vi "DAQ Test Program.vi"(8 "error in (no error)":errorcluster) -> (0 "error out":errorcluster)   [LabVIEW 2018, in "DAQ.lvlib"]
uses:
  DAQ.lvlib
  Acquisition/Acquisition State.ctl
  <vilib>/Platform/TimedLoop/XDataNode/timing_clust.ctl
  <vilib>/Platform/TimedLoop/XDataNode/nitl_modes.ctl
  <vilib>/Platform/TimedLoop/XDataNode/wakeup.ctl
  Acquisition/Task Cluster.ctl
  Acquisition/Hardware Configuration.ctl
  controls/Queue and Message Cluster.ctl
  support/Message Queue/Message Cluster.ctl
  support/Message Queue/Enqueue Message (Single).vi
  <vilib>/Platform/TimedLoop/XDataNode/XDataNode.xnode
  DAQ Write Folder/DAQ/DAQ Write.lvlib
  support/Message Queue/Message Queue.lvlib
  Report Generation/Report Generation.lvlib
  Acquisition/Acquisition Settings Dialog.vi
  support/Support Library.lvlib
  <vilib>/Platform/TimedLoop/XDataNode/XDNodeRunTimeDep.lvlib
panel:
  out "error IO":errorcluster
  out "Data Cluster 2":T1
  out "Task D-O Channels":string[][](array[string])
  in  "Stop Button":bool
  in  "Start Button":bool
  in  "Data Cluster":T1
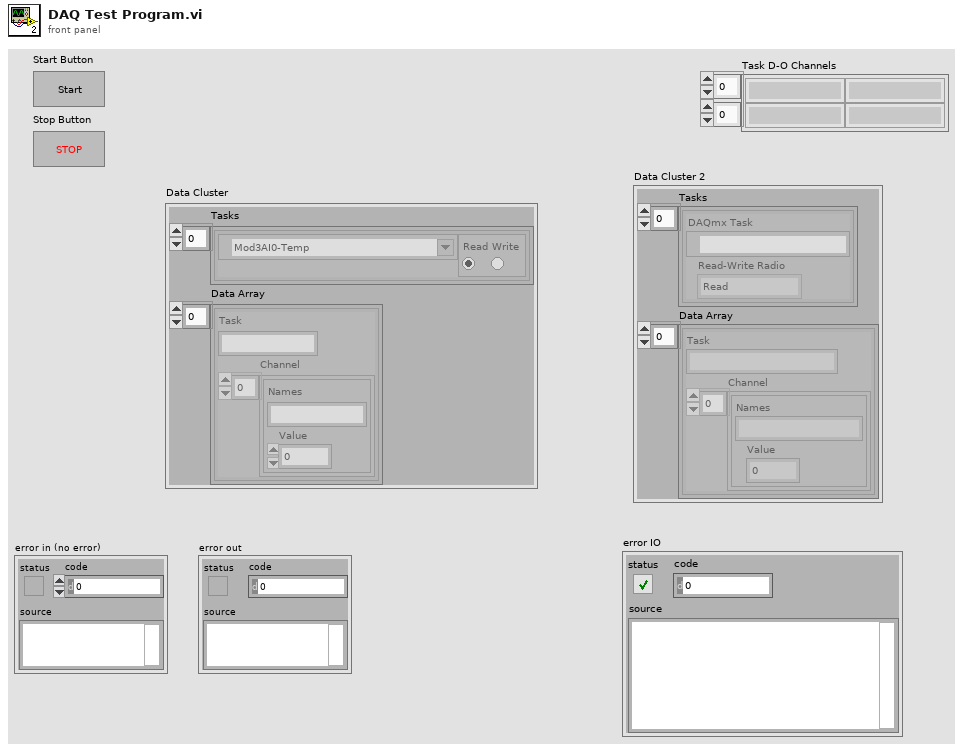
[diagram p1: front panel]
types:
  T1 = cluster{"Tasks":cluster{"DAQmx Task":refnum<k21>, "Read-Write Radio":enum32{"Read", "Write"}}[], "Data Array":cluster{"Task":string, "Channel":cluster{"Names":string, "Value":dbl}[]}[]}
  T2 = typedef "XDNodeRunTimeDep.lvlib/timing_clust.ctl" = cluster{"Expected End [f-1]":u64, "Actual End [f-1]":u64, "Finished Late? [f-1]":bool, "Expected End [i-1]":u64, "Actual End [i-1]":u64, "Finished Late? [i-1]":bool, "Expected Start [i]":u64, "Actual Start [i]":u64, "Expected Start [f]":u64, "Actual Start [f]":u64, "Source Name":string, "Structure Name":string, "Period":i64, "Deadline":i64, "Offset":i64, "Start":i64, "Priority":i32, "Timeout":i32, "Mode":T3, "Wakeup Reason":T4, "Error":errorcluster, "Source Type":string, "Secondary Source Type":string, "Global End Time":u64, "Global Start Time":u64, "Frame Duration":u64, "Iteration Duration":u64, "Assigned CPU":i32, "I/O Scan Engine Mode":u32}
  T3 = typedef "XDNodeRunTimeDep.lvlib/nitl_modes.ctl" = enum32{"No Change", "Process missed periods, maintain original phase", "Discard missed periods, maintain original phase", "Process missed periods, ignore original phase", "Discard missed periods, ignore original phase"}
  T4 = typedef "XDNodeRunTimeDep.lvlib/wakeup.ctl" = enum32{"Normal", "Aborted", "Asynchronous wakeup", "Timing source error", "Timed loop error", "Timeout"}
  T5 = typedef "Task Cluster.ctl" = cluster{"DAQmx Task":refnum<k21>, "Read-Write Radio":enum32{"Read", "Write"}}
  T6 = typedef "DAQ.lvlib/Hardware Configuration.ctl" = cluster{"Tasks Array":T5[]}
  T7 = typedef "DAQ.lvlib/DAQ Write.lvlib/Acquisition State.ctl" = enum16{"Idle", "Acquiring"}
  T8 = typedef "Queue and Message Cluster.ctl" = cluster{"return Message Queue":refnum<queue>, "Message":string, "Variant":variant}
  T9 = cluster{"DAQmx Task":refnum<k21>, "Read-Write Radio":enum32{"Read", "Write"}}[]
  T10 = cluster{"Task":string, "Channel":cluster{"Names":string, "Value":dbl}[]}[]
  T11 = typedef "Message Queue.lvlib/Message Cluster.ctl" = cluster{"Message":string, "Message Data":variant}
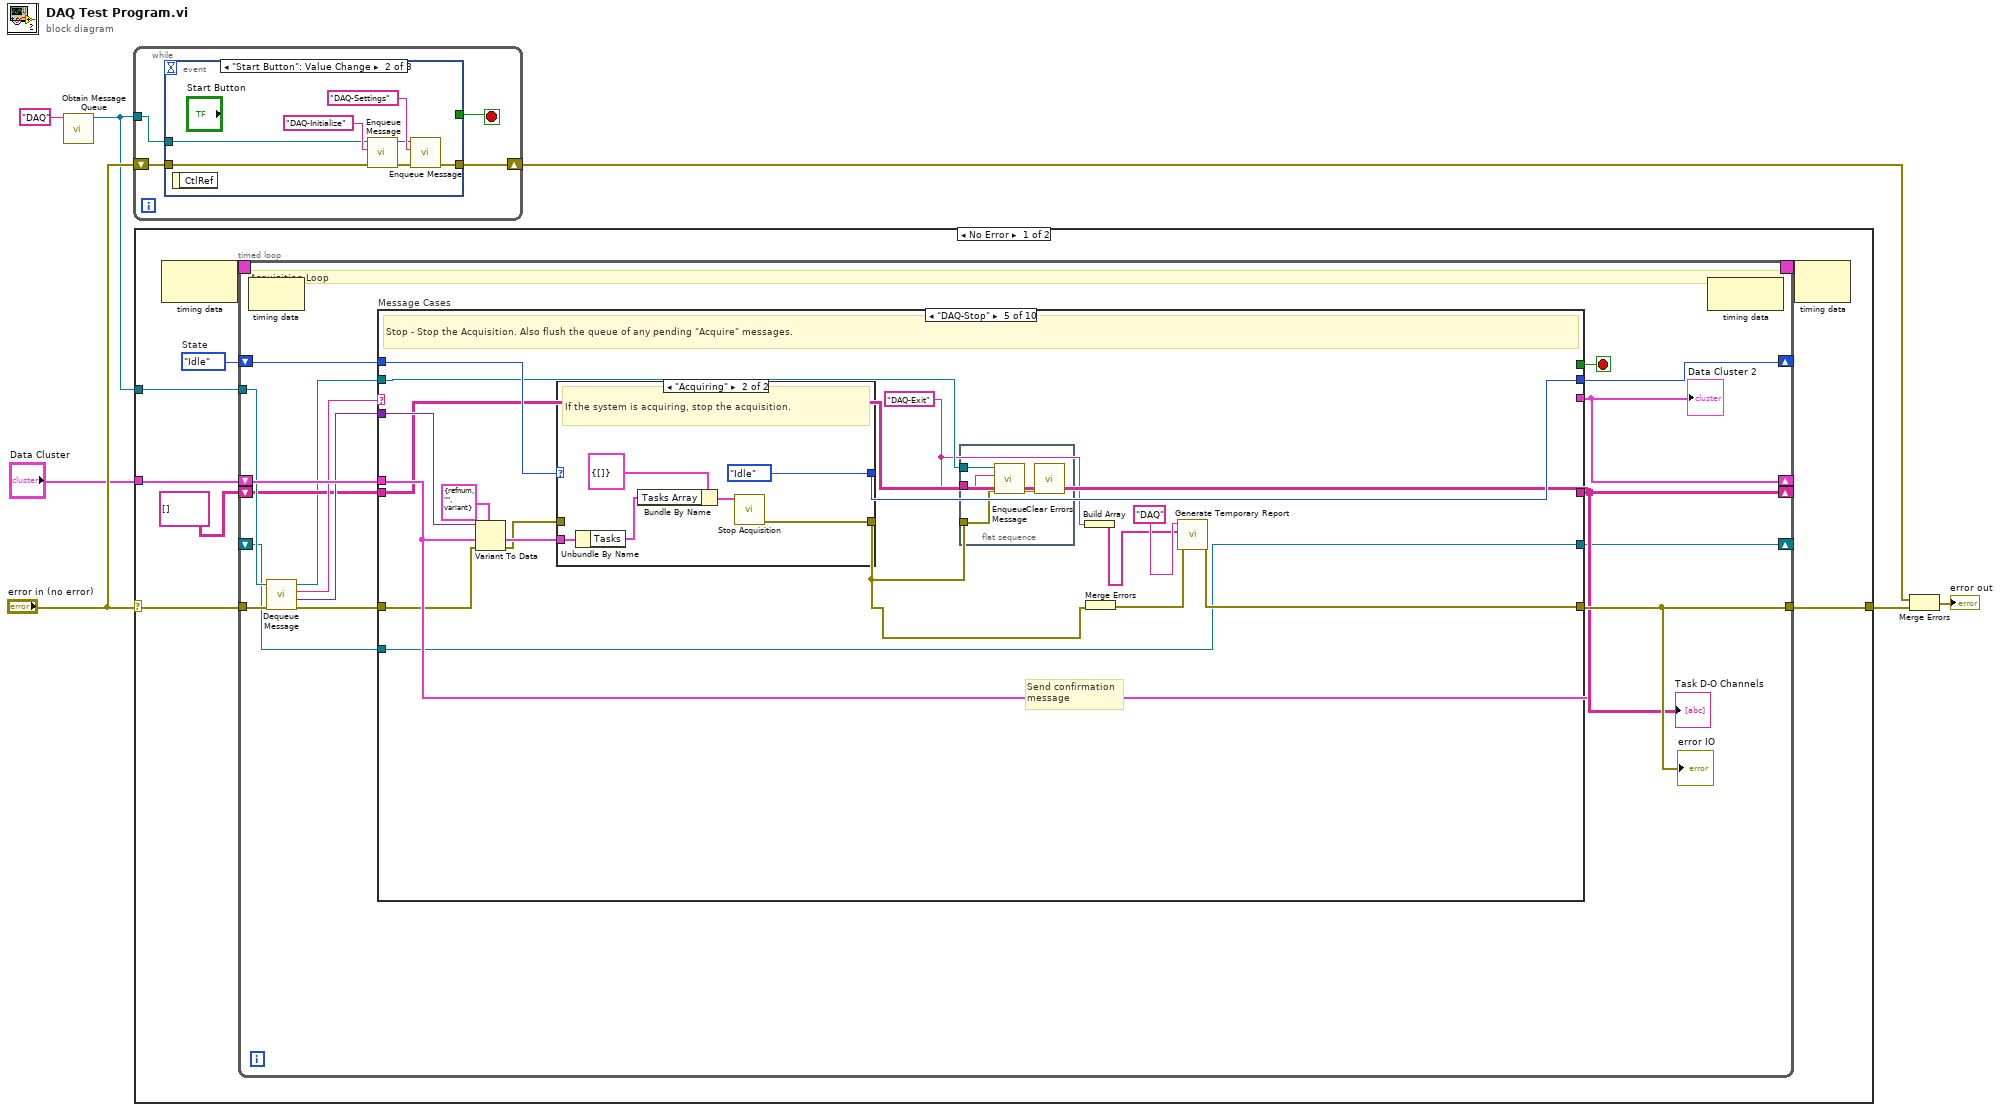
[diagram p0: block diagram]
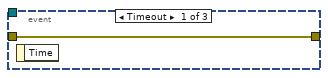
[diagram p2: hidden frame]
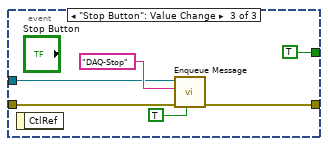
[diagram p3: hidden frame]
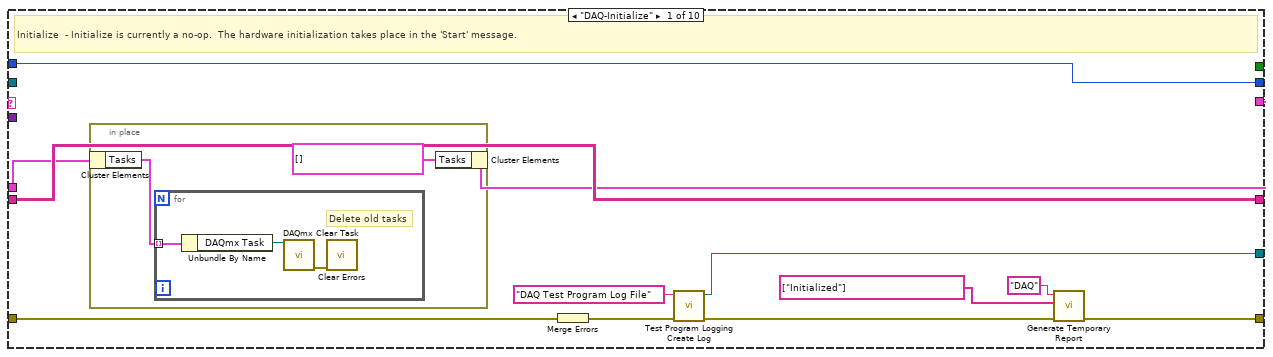
[diagram p4: hidden frame]
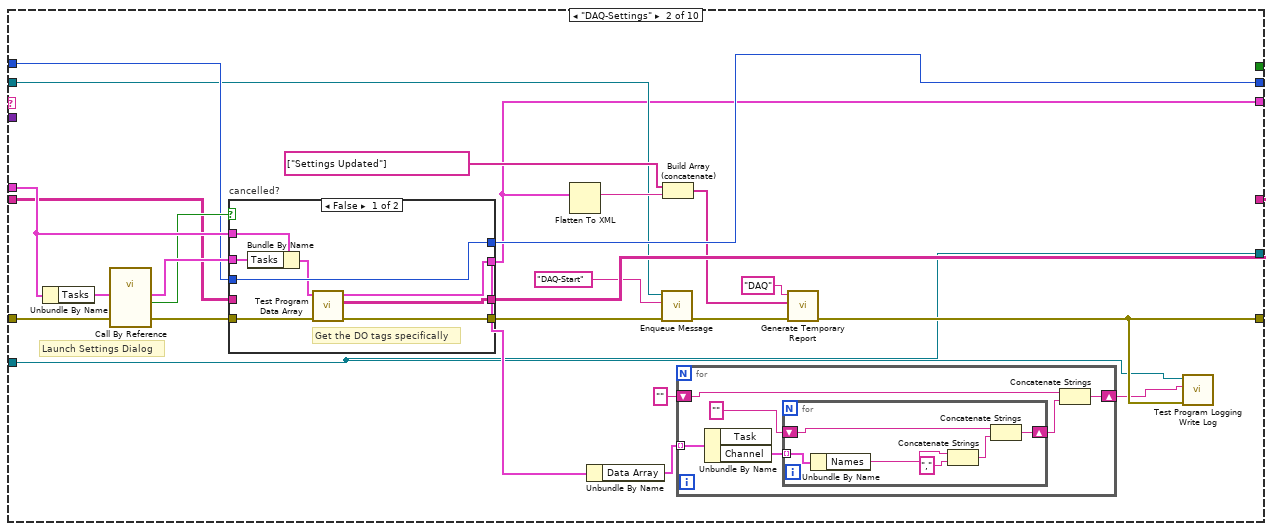
[diagram p5: hidden frame]
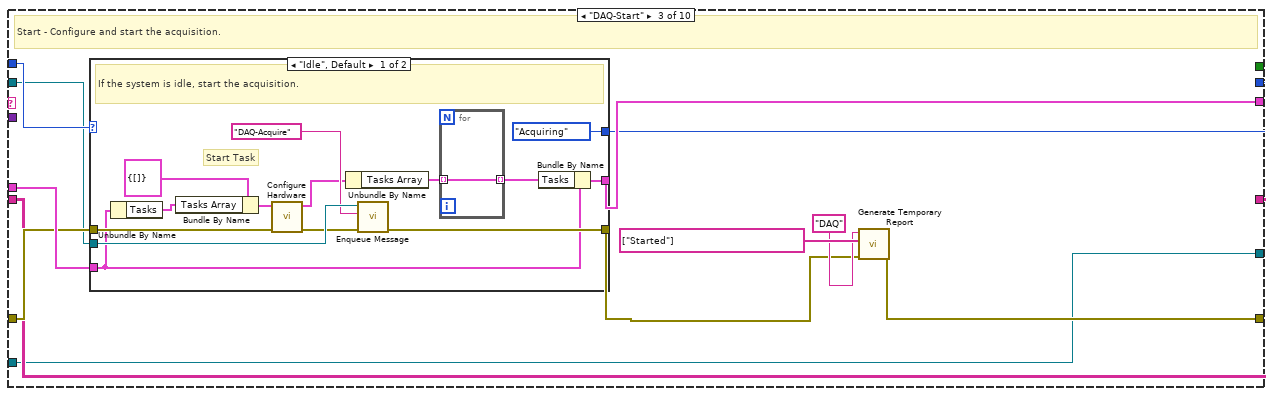
[diagram p7: hidden frame]
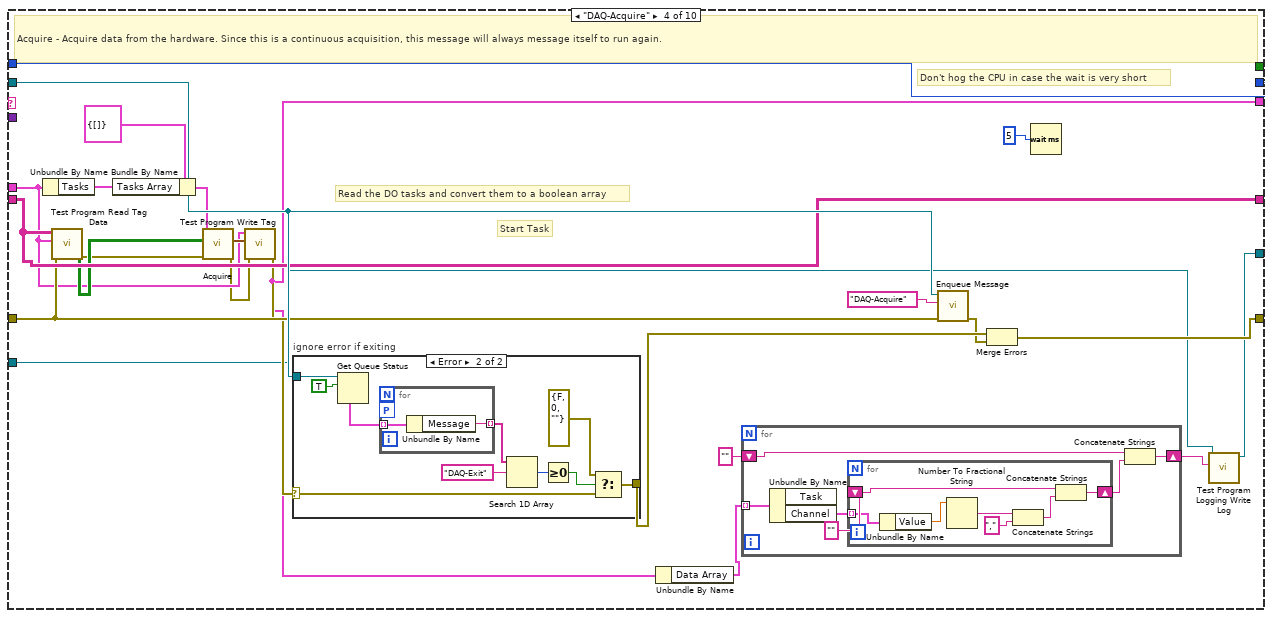
[diagram p9: hidden frame]
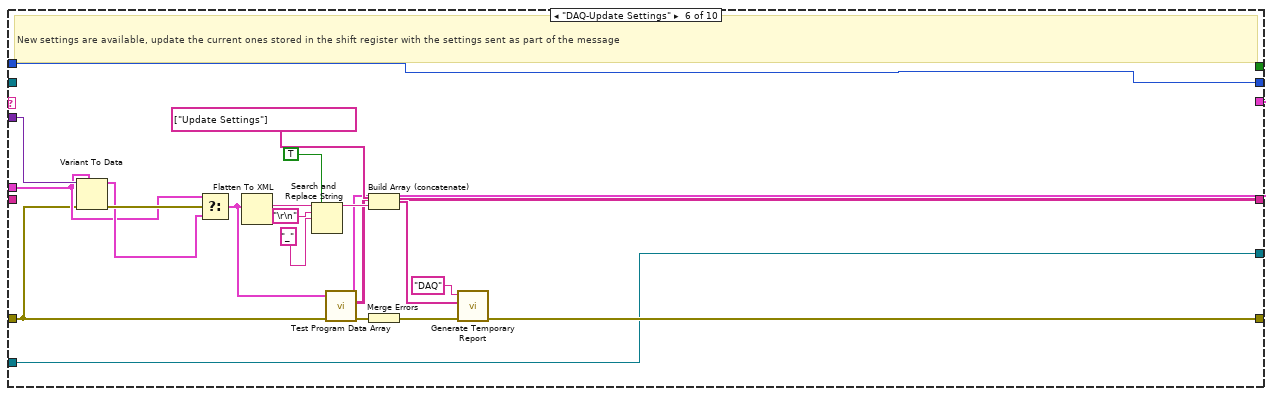
[diagram p12: hidden frame]
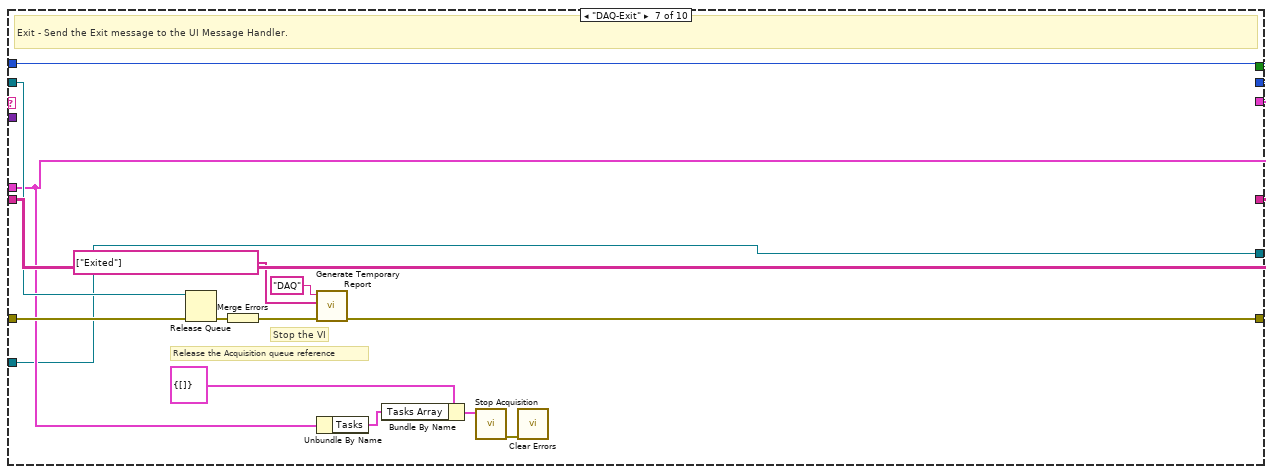
[diagram p13: hidden frame]
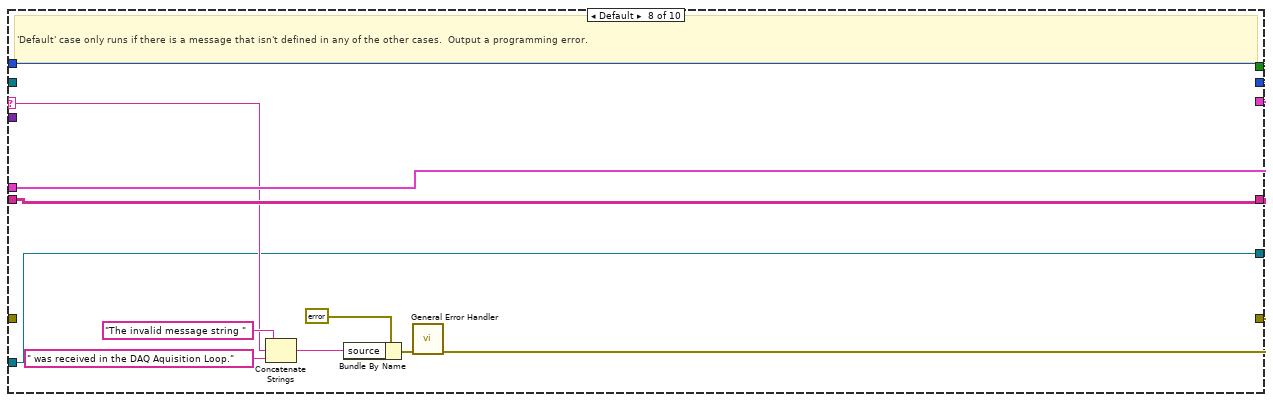
[diagram p14: hidden frame]
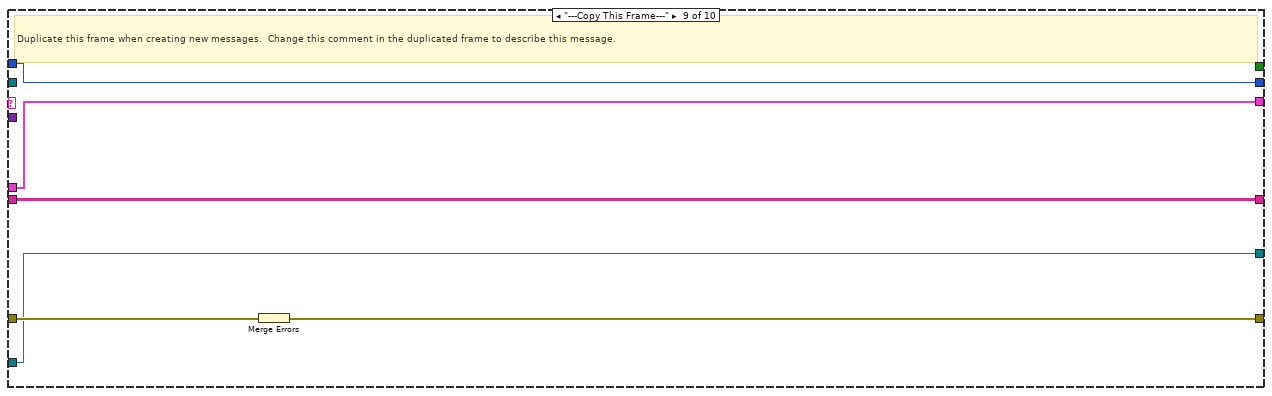
[diagram p15: hidden frame]
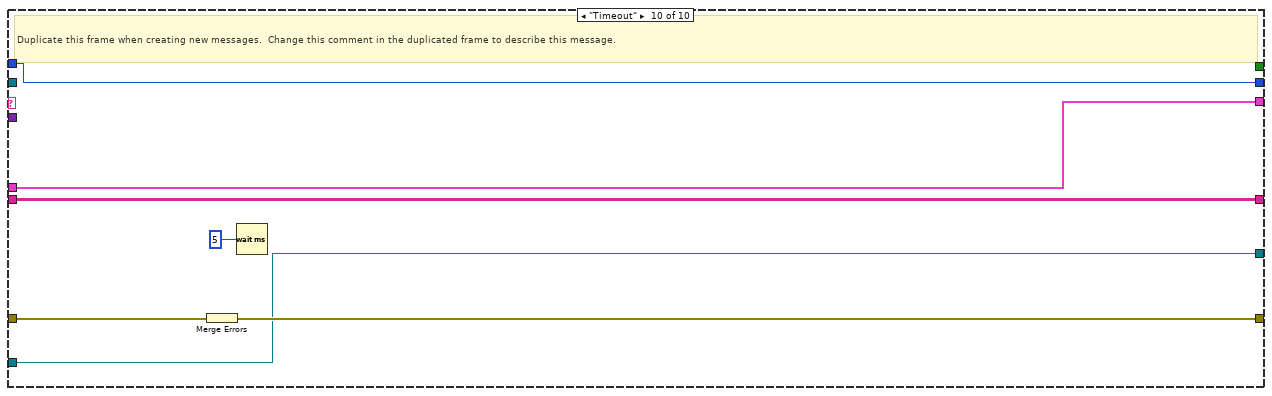
[diagram p16: hidden frame]
diagram:
  n1 = call "Obtain Message Queue.vi"("name (unnamed)"="DAQ") -> ("Message Queue"=w6:refnum<queue>)  [unwired: 9 in, 1 out]
  n2 = while {
    tunnel: w6 -> [w10]
    shift-right: [w9] -> w3
    shift-left: "error in (no error)" -> [w11]
    stop <- w8 stop-if-true
    n3 = event shown="[1] \"Start Button\": Value Change" {
      selector: _ -> [_ _ _]
      dyn-events: _ -> [_ _ _]
      timeout: _ -> [_ _ _]
      tunnel: w10 -> [_ w18 w24]
      tunnel: w11 -> [w12 w15 w23]
      tunnel: [w12 w13 w22] -> w9
      tunnel: [_ _ TRUE] -> w8
      event Timeout {
        n4 = event-data() -> ()  [unwired: 1 in, 1 out]
      }
      event "Start Button": Value Change {
        n5 = event-data() -> ()  [unwired: 1 in, 1 out]
        n6 = call-poly "Enqueue Message.vi"("error in (no error)"=w15, "Message"="DAQ-Initialize", "Message Queue"=w18) -> ("error out"=w14:errorcluster, "dup Message Queue"=w16:refnum<queue>)  [unwired: 7 in]
        n7 = call-poly "Enqueue Message.vi"("error in (no error)"=w14, "Message"="DAQ-Settings", "Message Queue"=w16) -> ("error out"=w13:errorcluster)  [unwired: 7 in, 1 out]
      }
      event "Stop Button": Value Change {
        n8 = event-data() -> ()  [unwired: 1 in, 1 out]
        n9 = call-poly "Enqueue Message.vi"("Priority Message? (F)"=TRUE, "error in (no error)"=w23, "Message"="DAQ-Stop", "Message Queue"=w24) -> ("error out"=w22:errorcluster)  [unwired: 6 in, 1 out]
      }
    }
  }
  n10 = case shown="No Error" "error in (no error)" {
    selector: "error in (no error)" -> [w32 w287]
    tunnel: [w33 w287] -> w4
    tunnel: "Data Cluster" -> [w29 _]
    tunnel: w6 -> [w28 _]
    frame No Error {
      w31 = Acquisition_State."Idle"  # State
      n11 = node-c288() -> (w27:T2)  [unwired: 1 in]
      n12 = timed-loop {
        tunnel: w28 -> [w43]
        shift-right: [w48] -> _
        shift-left: w29 -> [w49]
        shift-right: [w40] -> _
        shift-left: w31 -> [w41]
        shift-right: [w39] -> _
        shift-left: string[][] [] ("Task D-O Channels") -> [w38]
        tunnel: w32 -> [w46]
        tunnel: [w42] -> w33
        timing: w27 -> [_]
        timing-out: [_] -> w26
        shift-right: [w35] -> _
        shift-left: _ -> [w34]
        stop <- w47 stop-if-true
        # "Acquisition Loop"
        n13 = node-c288() -> ()  [unwired: 1 in, 1 out]
        n14 = call "Dequeue Message.vi"("error in (no error)"=w46, "Message Queue"=w43) -> ("error out"=w37:errorcluster, "Message Data"=w44:variant, "Message"=w45:string, "dup Message Queue"=w36:refnum<queue>)  [unwired: 6 in]
        n15 = case "Message Cases" shown="\"DAQ-Stop\"" w45 {
          selector: w45 -> [_ _ _ _ _ _ _ w263 _ _]
          tunnel: w37 -> [w63 w91 w127 w159 w206 w228 w260 _ w277 w284]
          tunnel: [w56 w72 w118 w164 w202 w239 w251 w264 w275 w282] -> w42
          tunnel: w49 -> [w60 w89 w128 w155 w212 w242 w248 w271 w276 w283]
          tunnel: [w59 w71 w126 w151 w212 w230 w248 w271 w276 w283] -> w48
          tunnel: [_ _ _ _ _ _ TRUE _ _ _] -> w47
          tunnel: w44 -> [_ _ _ _ w208 w245 _ _ _ _]
          tunnel: w41 -> [w62 w84 w125 w170 w211 w241 w258 w270 w274 w281]
          tunnel: [w62 w83 w124 w170 w210 w241 w258 w270 w274 w281] -> w40
          tunnel: [w61 w86 w123 w160 w204 w229 w256 w269 w273 w280] -> w39
          tunnel: w38 -> [w61 w85 w123 w160 w204 _ w256 w269 w273 w280]
          tunnel: w36 -> [_ w77 w122 w165 w200 _ w255 _ _ _]
          tunnel: [w52 w70 w117 w147 w197 w225 w246 w262 w272 w278] -> w35
          tunnel: w34 -> [_ w70 w117 w148 w197 w225 w246 w262 w272 w278]
          frame "DAQ-Initialize" {
            # "Initialize  - Initialize is currently a no-op.  The hardware initialization takes place in the 'Start' message."
            n16 = in-place {
              n17 = in-place-cluster #1(w60) -> ("Tasks"=w65:T9)
              n18 = for {
                tunnel: w65 -> [w68] mode=indexing
                # "Delete old tasks"
                n19 = Unbundle By Name(w68) -> ("DAQmx Task"=w67:refnum<k21>)
                n20 = call <vilib>:"DAQmx Clear Task.vi"("task in"=w67) -> ("error out"=w66:errorcluster)  [unwired: 14 in]
                n21 = call <vilib>:"Clear Errors.vi"("error in (no error)"=w66) -> ()  [unwired: 5 in, 2 out]
              }
              n22 = in-place-cluster #1("Tasks"=T5[] []) -> (w59:T1)
            }
            n23 = Merge Errors(w63) -> (w55:errorcluster)
            n24 = call "Test Program Logging Create Log.vi"("error in"=w55, "string"="DAQ Test Program Log File") -> ("error out"=w54:errorcluster, "refnum out"=w52:refnum<file>)  [unwired: 8 in]
            n25 = call "Generate Temporary Report.vi"("error in (no error)"=w54, "Line of Events"=string[] ["Initialized"], "Module Name"="DAQ") -> ("error out"=w56:errorcluster)  [unwired: 8 in]
          }
          frame "DAQ-Settings" {
            # "Launch Settings Dialog"
            n26 = Unbundle By Name(w89) -> ("Tasks"=w90:T9)
            n27 = call-by-ref "?"("error in (no error)"=w91, "Tasks in"=w90) -> ("error out"=w87:errorcluster, "cancelled"=w88:bool, "Tasks out"=w92:T5[])  [unwired: 9 in, 2 out]
            n28 = case "cancelled?" shown="False" w88 {
              tunnel: w92 -> [w111 _]
              tunnel: w89 -> [w112 w113]
              tunnel: w87 -> [w108 w116]
              tunnel: [w107 w116] -> w76
              tunnel: [w106 w115] -> w86
              tunnel: w85 -> [_ w115]
              tunnel: [w110 w114] -> w83
              tunnel: w84 -> [w110 w114]
              tunnel: [w105 w113] -> w71
              frame False {
                # "Get the DO tags specifically"
                n29 = Bundle By Name(cluster=w112, "Tasks"=w111) -> (w109:T1)
                n30 = call "Test Program Data Array.vi"("error in (no error)"=w108, "Data Cluster in"=w109) -> ("error out"=w107:errorcluster, "Task D-O Channels"=w106:string[][], "Data Cluster out"=w105:T1)  [unwired: 7 in]
              }
              frame True {
              }
            }
            n31 = Flatten To XML(anything=w71) -> (xml string=w79:string)
            n32 = Unbundle By Name(w71) -> ("Data Array"=w74:T10)
            n33 = call-poly "Enqueue Message.vi"("error in (no error)"=w76, "Message"="DAQ-Start", "Message Queue"=w77) -> ("error out"=w75:errorcluster)  [unwired: 7 in, 1 out]
            n34 = Build Array (concatenate)(string[] ["Settings Updated"] ("Line of Events"), w79) -> (w80:string[])
            n35 = for {
              tunnel: w74 -> [w98] mode=indexing
              shift-right: [w95] -> w69
              shift-left: "" -> [w94]
              n36 = Unbundle By Name(w98) -> ("Channel"=w97:cluster{"Names":string, "Value":dbl}[])  [unwired: 1 out]
              n37 = for {
                tunnel: w97 -> [w104] mode=indexing
                shift-right: [w100] -> w96
                shift-left: "" -> [w102]
                n38 = Unbundle By Name(w104) -> ("Names"=w99:string)
                n39 = Concatenate Strings(w99, "," ("string")) -> (w101:string)
                n40 = Concatenate Strings(w102, w101) -> (w100:string)
              }
              n41 = Concatenate Strings(w94, w96) -> (w95:string)
            }
            n42 = call "Generate Temporary Report.vi"("error in (no error)"=w75, "Line of Events"=w80, "Module Name"="DAQ") -> ("error out"=w72:errorcluster)  [unwired: 8 in]
            n43 = call "Test Program Logging Write Log.vi"("error in"=w72, "text"=w69, "Test Program Log File"=w70) -> ()  [unwired: 7 in, 2 out]
          }
          frame "DAQ-Start" {
            # "Start - Configure and start the acquisition."
            n44 = case shown="\"Idle\", Default" w125 {
              selector: w125 -> [_ w144]
              tunnel: [w139 w146] -> w119
              tunnel: w128 -> [w131 w145]
              tunnel: w127 -> [w141 w146]
              tunnel: w122 -> [w140 _]
              tunnel: [w130 w145] -> w126
              tunnel: [Acquisition_State."Acquiring" ("State") w144] -> w124
              frame "Idle", Default {
                # "Start Task"
                # "If the system is idle, start the acquisition."
                n45 = Unbundle By Name(w131) -> ("Tasks"=w135:T9)
                n46 = Bundle By Name(cluster=T6 {"Tasks Array"=[]} ("Hardware Resources in"), "Tasks Array"=w135) -> (w134:T6)
                n47 = call "Configure Hardware.vi"("error in (no error)"=w141, "Hardware Resources in"=w134) -> ("error out"=w137:errorcluster, "Hardware Resources out"=w133:T6)  [unwired: 8 in]
                n48 = Unbundle By Name(w133) -> ("Tasks Array"=w132:T5[])
                n49 = call-poly "Enqueue Message.vi"("error in (no error)"=w137, "Message"="DAQ-Acquire", "Message Queue"=w140) -> ("error out"=w139:errorcluster)  [unwired: 7 in, 1 out]
                n50 = for {
                  tunnel: w132 -> [w143] mode=indexing
                  tunnel: [w143] -> w129 mode=indexing
                }
                n51 = Bundle By Name(cluster=w131, "Tasks"=w129) -> (w130:T1)
              }
              frame "Acquiring" {
                # "The system is already acquiring. Ignore the \"Start\" message."
              }
            }
            n52 = call "Generate Temporary Report.vi"("error in (no error)"=w119, "Line of Events"=string[] ["Started"], "Module Name"="DAQ") -> ("error out"=w118:errorcluster)  [unwired: 8 in]
          }
          frame "DAQ-Acquire" {
            # "Read the DO tasks and convert them to a boolean array"
            # "Start Task"
            # "Don't hog the CPU in case the wait is very short"
            # "Acquire - Acquire data from the hardware. Since this is a continuous acquisition, this message will always message itself to run again."
            n53 = Unbundle By Name(w155) -> ("Tasks"=w162:T9)
            n54 = call "Test Program Read Tag Data.vi"("error in (no error)"=w159, "Data Cluster"=w155, "Task D-O Channels"=w160) -> ("error out"=w157:errorcluster, "Array"=w158:bool[][])  [unwired: 7 in]
            n55 = Bundle By Name(cluster=T6 {"Tasks Array"=[]} ("Hardware Resources in"), "Tasks Array"=w162) -> (w161:T6)
            n56 = call "Acquire.vi"("error in (no error)"=w157, "Digital Write Status"=w158, "Hardware Resources in"=w161) -> ("error out"=w153:errorcluster, "data"=w156:waveform(dbl)[])  [unwired: 6 in, 1 out]
            n57 = call "Test Program Write Tag.vi"("error in (no error)"=w153, "data"=w156, "Data Cluster"=w155) -> ("error out"=w154:errorcluster, "Data Cluster 3"=w151:T1)  [unwired: 5 in, 2 out]
            n58 = case "ignore error if exiting" shown="Error" w154 {
              selector: w154 -> [w184 w187]
              tunnel: w165 -> [_ w194]
              tunnel: [w184 w186] -> w168
              frame No Error {
              }
              frame Error {
                n59 = Get Queue Status(queue=w194, return elements? (F)=TRUE) -> (elements=w191:T11[])  [unwired: 1 in, 7 out]
                n60 = for {
                  tunnel: w191 -> [w196] mode=indexing
                  tunnel: [w195] -> w190 mode=indexing
                  workers-P: _ -> [_]
                  n61 = Unbundle By Name(w196) -> ("Message"=w195:string)
                }
                n62 = Search 1D Array(1D array=w190, element="DAQ-Exit") -> (index of element=w189:i32)  [unwired: 1 in]
                n63 = Greater Or Equal To 0?(x=w189) -> (x >= 0?=w188:bool)
                n64 = Select(t=errorcluster {"status"=FALSE, "code"=0, "source"=""}, s=w188, f=w187) -> (s? t:f=w186:errorcluster)
              }
            }
            n65 = Unbundle By Name(w151) -> ("Data Array"=w152:T10)
            n66 = for {
              tunnel: w152 -> [w176] mode=indexing
              shift-right: [w173] -> w149
              shift-left: "" -> [w172]
              n67 = Unbundle By Name(w176) -> ("Channel"=w175:cluster{"Names":string, "Value":dbl}[])  [unwired: 1 out]
              n68 = for {
                tunnel: w175 -> [w183] mode=indexing
                shift-right: [w179] -> w174
                shift-left: "" -> [w181]
                n69 = Unbundle By Name(w183) -> ("Value"=w177:dbl)
                n70 = Number To Fractional String(number=w177) -> (F-format string=w178:string)  [unwired: 3 in]
                n71 = Concatenate Strings(w178, "," ("string")) -> (w180:string)
                n72 = Concatenate Strings(w181, w180) -> (w179:string)
              }
              n73 = Concatenate Strings(w172, w174) -> (w173:string)
            }
            n74 = call-poly "Enqueue Message.vi"("error in (no error)"=w159, "Message"="DAQ-Acquire", "Message Queue"=w165) -> ("error out"=w167:errorcluster)  [unwired: 7 in, 1 out]
            n75 = Merge Errors(w168, w167) -> (w164:errorcluster)
            n76 = Wait (ms)(milliseconds to wait=u32 5) -> ()  [unwired: 1 out]
            n77 = call "Test Program Logging Write Log.vi"("text"=w149, "Test Program Log File"=w148) -> ("refnum out"=w147:refnum<file>)  [unwired: 8 in, 1 out]
          }
          frame "DAQ-Stop" {
            w199 = "DAQ-Exit" ("Message")
            # "Send confirmation\nmessage"
            # "Stop - Stop the Acquisition. Also flush the queue of any pending \"Acquire\" messages."
            n78 = Variant To Data(error in=w206, type=T8 {"return Message Queue"=refnum, "Message"="", "Variant"=variant} ("Queue and Message"), Variant=w208) -> (error out=w207:errorcluster)  [unwired: 1 out]
            n79 = case shown="\"Acquiring\"" w211 {
              selector: w211 -> [w218 _]
              tunnel: w207 -> [w217 _]
              tunnel: w212 -> [_ w220]
              tunnel: [w218 Acquisition_State."Idle" ("State")] -> w210
              tunnel: [w217 w223] -> w205
              frame "Idle", Default {
                # "The system is already idle. Ignore the \"Stop\" message."
              }
              frame "Acquiring" {
                # "If the system is acquiring, stop the acquisition."
                n80 = Unbundle By Name(w220) -> ("Tasks"=w222:T9)
                n81 = Bundle By Name(cluster=T6 {"Tasks Array"=[]} ("Hardware Resources in"), "Tasks Array"=w222) -> (w219:T6)
                n82 = call "Stop Acquisition.vi"("Hardware Resources in"=w219) -> ("error out"=w223:errorcluster)  [unwired: 10 in]
              }
            }
            n83 = flat-sequence {
              tunnel: w200 -> [w216]
              tunnel: w199 -> [w215]
              tunnel: w205 -> [w213]
              frame #0 {
                n84 = call-poly "Enqueue Message.vi"("error in (no error)"=w213, "Message"=w215, "Message Queue"=w216) -> ("error out"=w214:errorcluster)  [unwired: 7 in, 1 out]
                n85 = call <vilib>:"Clear Errors.vi"("error in (no error)"=w214) -> ()  [unwired: 5 in, 2 out]
              }
            }
            n86 = Build Array(w199) -> (w198:string[])
            n87 = Merge Errors(w205) -> (w201:errorcluster)
            n88 = call "Generate Temporary Report.vi"("error in (no error)"=w201, "Line of Events"=w198, "Module Name"="DAQ") -> ("error out"=w202:errorcluster)  [unwired: 8 in]
          }
          frame "DAQ-Update Settings" {
            # "New settings are available, update the current ones stored in the shift register with the settings sent as part of the message"
            n89 = Variant To Data(error in=w228, type=w242, Variant=w245) -> (data=w243:T1, error out=w244:errorcluster)
            n90 = Select(t=w242, s=w244, f=w243) -> (s? t:f=w231:T1)
            n91 = Flatten To XML(anything=w231) -> (xml string=w233:string)
            n92 = Search and Replace String(replace all?=TRUE ("replace all? (F)"), input string=w233, search string="\r\n", replace string="_" ("replace string (\"\")")) -> (result string=w232:string)  [unwired: 4 in, 3 out]
            n93 = call "Test Program Data Array.vi"("error in (no error)"=w228, "Data Cluster in"=w231) -> ("error out"=w226:errorcluster, "Task D-O Channels"=w229:string[][], "Data Cluster out"=w230:T1)  [unwired: 7 in]
            n94 = Build Array (concatenate)(string[] ["Update Settings"] ("Line of Events"), w232) -> (w237:string[])
            n95 = Merge Errors(w226) -> (w227:errorcluster)
            n96 = call "Generate Temporary Report.vi"("error in (no error)"=w227, "Line of Events"=w237, "Module Name"="DAQ") -> ("error out"=w239:errorcluster)  [unwired: 8 in]
          }
          frame "DAQ-Exit" {
            # "Release the Acquisition queue reference"
            # "Stop the VI"
            # "Exit - Send the Exit message to the UI Message Handler."
            n97 = Release Queue(queue=w255, error in (no error)=w260) -> (error out=w259:errorcluster)  [unwired: 1 in, 2 out]
            n98 = Merge Errors(w259) -> (w252:errorcluster)
            n99 = call "Generate Temporary Report.vi"("error in (no error)"=w252, "Line of Events"=string[] ["Exited"], "Module Name"="DAQ") -> ("error out"=w251:errorcluster)  [unwired: 8 in]
            n100 = Unbundle By Name(w248) -> ("Tasks"=w250:T9)
            n101 = Bundle By Name(cluster=T6 {"Tasks Array"=[]} ("Hardware Resources in"), "Tasks Array"=w250) -> (w247:T6)
            n102 = call "Stop Acquisition.vi"("Hardware Resources in"=w247) -> ("error out"=w257:errorcluster)  [unwired: 10 in]
            n103 = call <vilib>:"Clear Errors.vi"("error in (no error)"=w257) -> ()  [unwired: 5 in, 2 out]
          }
          frame Default {
            # "'Default' case only runs if there is a message that isn't defined in any of the other cases.  Output a programming error."
            n104 = Concatenate Strings("The invalid message string " ("string"), w263, " was received in the DAQ Aquisition Loop." ("string")) -> (w265:string)
            n105 = Bundle By Name(cluster=errorcluster {"status"=TRUE, "code"=1, "source"=""} ("error constant"), "source"=w265) -> (w264:errorcluster)
            n106 = call <vilib>:"General Error Handler.vi"("error in (no error)"=w264) -> ()  [unwired: 10 in, 5 out]
          }
          frame "---Copy This Frame---" {
            # "Duplicate this frame when creating new messages.  Change this comment in the duplicated frame to describe this message."
            n107 = Merge Errors(w277) -> (w275:errorcluster)
          }
          frame "Timeout" {
            # "Duplicate this frame when creating new messages.  Change this comment in the duplicated frame to describe this message."
            n108 = Merge Errors(w284) -> (w282:errorcluster)
            n109 = Wait (ms)(milliseconds to wait=u32 5) -> ()  [unwired: 1 out]
          }
        }
        "Task D-O Channels" <- w39
        "Data Cluster 2" <- w48
        "error IO" <- w42
        n110 = node-c288() -> ()  [unwired: 1 in, 1 out]
      }
      n111 = node-c288(w26) -> ()  [unwired: 1 out]
    }
    frame Error {
    }
  }
  n112 = Merge Errors(w3, w4) -> (→"error out":errorcluster)
